vi "Write Port.vi"(2 "Timeout":i16, 8 "error in (no error)":errorcluster, 9 "Port":T1="Mod6\\Port1", 10 "Data":u8, 11 "MPU in":refnum<class "MPU.lvclass">) -> (0 "error out":errorcluster, 1 "Timeouted":bool, 3 "MPU out":refnum<class "MPU.lvclass">)   [LabVIEW 2018, in "Modbus_Processing_Unit.lvlib" / "MPU.lvclass"]
uses:
  MPU.lvclass
  PortType.ctl
  <vilib>/rvi/eio/common/nirviEmuTemplateMethod_errors.vi
  <vilib>/eio/EIONode/EIONode.xnode
  <vilib>/eio/EIOMethodNode/EIOMethodNode.xnode
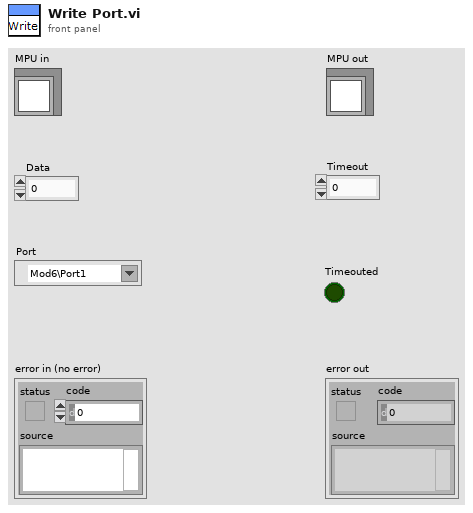
[diagram p1: front panel]
types:
  T1 = typedef "PortType.ctl" = refnum<k21>
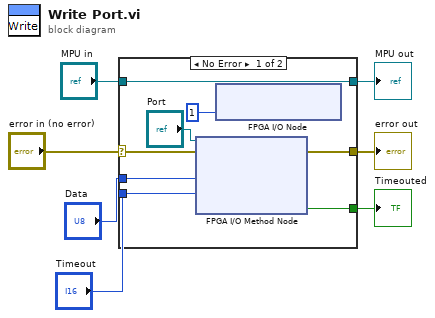
[diagram p0: block diagram]
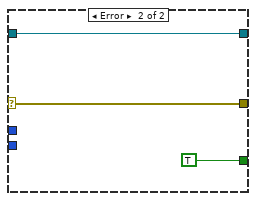
[diagram p2: hidden frame]
diagram:
  n1 = case shown="No Error" "error in (no error)" {
    selector: "error in (no error)" -> [w12 w18]
    tunnel: [w11 w18] -> w6
    tunnel: [w10 w17] -> w4
    tunnel: "MPU in" -> [w10 w17]
    tunnel: "Data" -> [w15 _]
    tunnel: "Timeout" -> [w14 _]
    tunnel: [w13 TRUE ("Timed Out")] -> w1
    frame No Error {
      n2 = xnode "FPGA I/O Method Node"("error in"=w12, "FPGA I/O In"="Port", "Data"=w15, "Timeout (ms)"=w14) -> ("error out"=w11:errorcluster, "Timed Out"=w13:bool)  [unwired: 1 out]
      n3 = xnode "FPGA I/O Node"("USER FPGA LED"=u8 1) -> ()  [unwired: 1 in, 1 out]
    }
    frame Error {
    }
  }
  "error out" <- w6
  "MPU out" <- w4
  "Timeouted" <- w1
